vi "故障码字段定义.vi"(11 "故障代码":u16) -> (3 "报警":T1)   [LabVIEW 2016, in "斯坦道总氮V2.lvlib"]
uses:
  Alarm interface/Alarm interface.lvlib
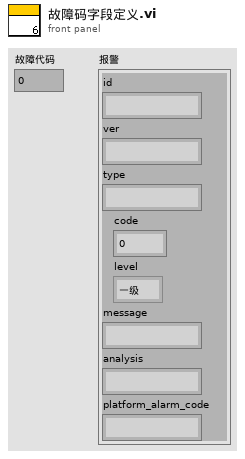
[diagram p1: front panel]
types:
  T1 = cluster{"id":string, "ver":string, "type":string, "code":u16, "level":enum16{"一级", "二级", "三级"}, "message":string, "analysis":string, "platform_alarm_code":string}
  T2 = cluster{"id":string, "ver":string, "type":enum16{"Alarm", "Fault"}, "code":u16}
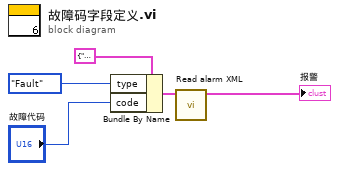
[diagram p0: block diagram]
diagram:
  n1 = Bundle By Name(cluster=T2 {"id"="斯坦道营养盐", "ver"="A", "type"=enum."Alarm", "code"=1} ("筛选输入"), "type"=enum16{"Alarm", "Fault"}."Fault", "code"="故障代码") -> (w4:T2)
  n2 = call "Read alarm XML.vi"("筛选输入"=w4) -> ("报警"=→"报警":T1)  [unwired: 9 in]
